vi "convertEntryParaTableToArray.vi"(8 "error in":errorcluster, 11 "entryParaTbl":string[][](array[string])) -> (0 "error out":errorcluster, 3 "contArr":string[](array[string]))   [LabVIEW 2010]
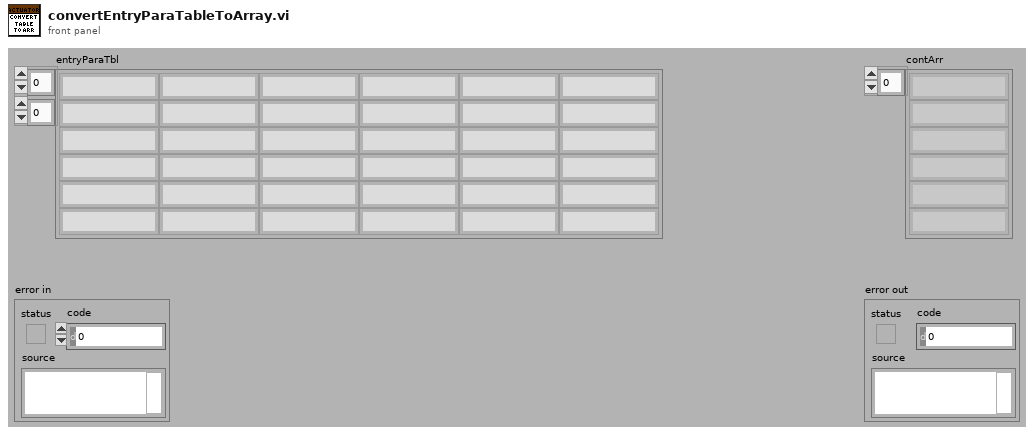
[diagram p1: front panel]
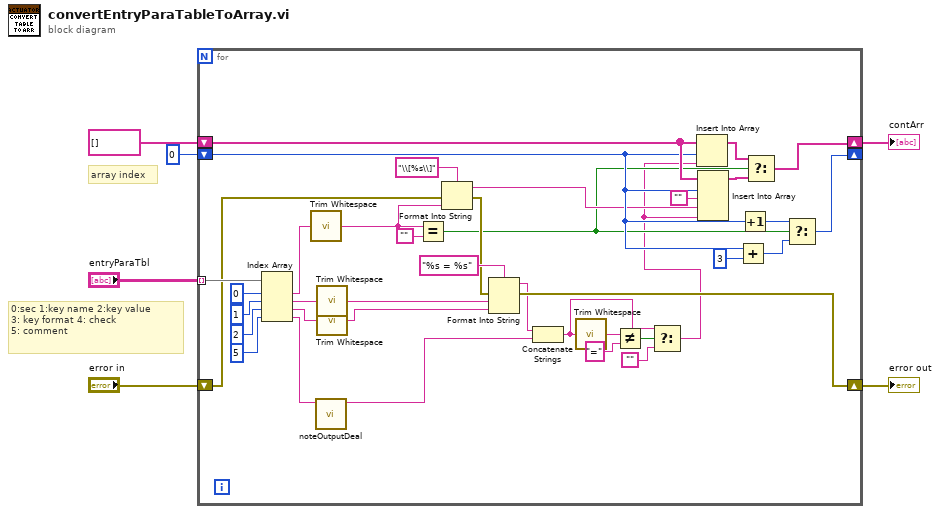
[diagram p0: block diagram]
diagram:
  # "0:sec 1:key name 2:key value \n3: key format 4: check \n5: comment"
  # "array index"
  n1 = for {
    tunnel: "entryParaTbl" -> [w43] mode=indexing
    shift-right: [w31] -> w2
    shift-left: string[] [] ("Value") -> [w33]
    shift-right: [w28] -> w1
    shift-left: "error in" -> [w29]
    shift-right: [w30] -> _
    shift-left: 0 ("input 1") -> [w32]
    n2 = Index Array(array=w43, index #1=0 ("index"), index #2=1 ("index"), index #3=2 ("index"), index #4=5 ("index")) -> (element #1=w38:string, element #2=w39:string, element #3=w37:string, element #4=w35:string)
    n3 = call <vilib>:"Trim Whitespace.vi"("string"=w38) -> ("trimmed string"=w36:string)  [unwired: 1 in]
    n4 = call "noteOutputDeal.vi"("note in editor"=w35) -> ("note output"=w34:string)  [unwired: 10 in]
    n5 = call <vilib>:"Trim Whitespace.vi"("string"=w39) -> ("trimmed string"=w14:string)  [unwired: 1 in]
    n6 = call <vilib>:"Trim Whitespace.vi"("string"=w37) -> ("trimmed string"=w13:string)  [unwired: 1 in]
    n7 = Equal?(x=w36, y="") -> (x = y?=w18:bool)
    n8 = Format Into String(format string="\\[%s\\]", error in=w29, w36) -> (resulting string=w20:string, error out=w22:errorcluster)  [unwired: 1 in]
    n9 = Format Into String(format string="%s = %s", error in=w22, w14, w13) -> (resulting string=w25:string, error out=w28:errorcluster)  [unwired: 1 in]
    n10 = Concatenate Strings(w25, w34) -> (w9:string)
    n11 = call <vilib>:"Trim Whitespace.vi"("string"=w9) -> ("trimmed string"=w12:string)  [unwired: 1 in]
    n12 = Not Equal?(x=w12, y="=") -> (x != y?=w10:bool)
    n13 = Select(t=w9, s=w10, f="") -> (s? t:f=w7:string)
    n14 = Insert Into Array(array=w33, index=w32, new element=w7) -> (w24:string[])
    n15 = Insert Into Array(array=w33, index=w32, new element #1="", new element #2=w20, new element #3=w7) -> (w19:string[])
    n16 = Add(x=w32, y=3) -> (x+y=w16:i32)
    n17 = Increment(x=w32) -> (x+1=w17:i32)
    n18 = Select(t=w24, s=w18, f=w19) -> (s? t:f=w31:string[])
    n19 = Select(t=w17, s=w18, f=w16) -> (s? t:f=w30:i32)
  }
  "contArr" <- w2
  "error out" <- w1
